vi "Init.vi"(1 "AI Range (V)":cluster{"AImin":dbl, "AImax":dbl}={"AImin"=-10.0, "AImax"=10.0}, 2 "Repetitions":u32, 5 "Pixel Dwell time (s)":dbl format="%#_6p", 7 "Trigger terminal":tag, 9 "AI Channels":tag, 11 "error in":errorcluster, 12 "input terminal configuration":i32(ring)=-1 items=["default"=-1, "RSE"=10083, "NRSE"=10078, "Differential"=10106, "Pseudodifferential"=12529]) -> (4 "AI Task out":refnum<k21>, 15 "error out":errorcluster)   [LabVIEW 2025]
uses:
  <vilib>/DAQmx/create/channels.llb/DAQmx Create Channel (AI-Voltage-Basic).vi
  <vilib>/DAQmx/configure/timing.llb/DAQmx Timing (Sample Clock).vi
  <vilib>/DAQmx/configure/trigger.llb/DAQmx Start Trigger (Digital Edge).vi
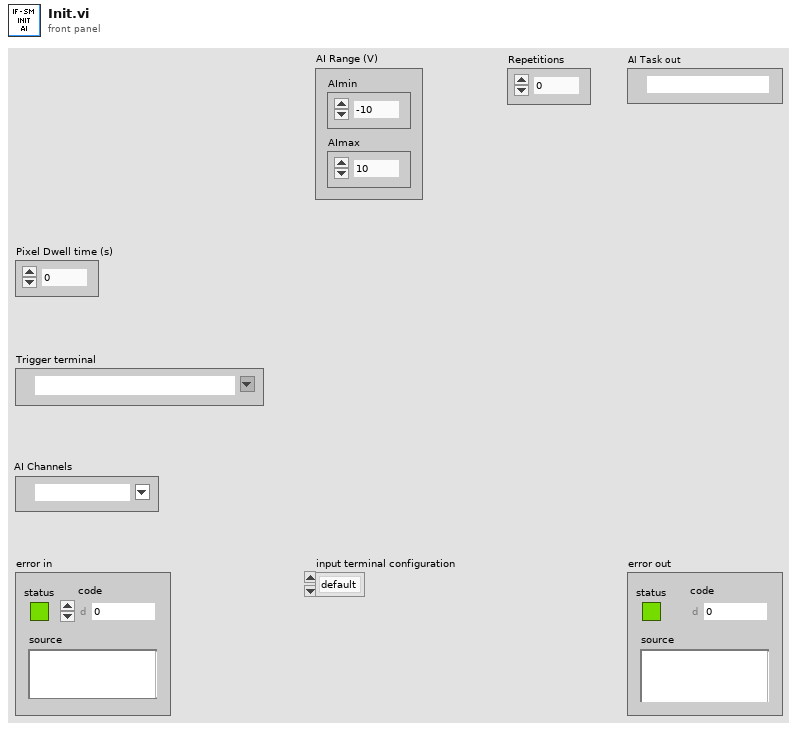
[diagram p1: front panel]
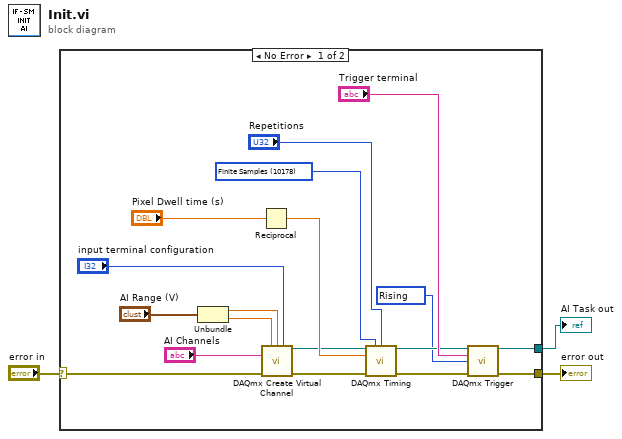
[diagram p0: block diagram]
diagram:
  n1 = case shown="No Error" "error in" {
    selector: "error in" -> [w4 w22]
    tunnel: [w21 w22] -> w3
    tunnel: [w5 _] -> w2
    frame No Error {
      w9 = 10280 items=["Rising"=10280, "Falling"=10171] ("edge")
      w15 = 10178 items=["Finite Samples"=10178, "Continuous Samples"=10123] ("sample mode")
      n2 = Unbundle("AI Range (V)") -> ("AImin"=w7:dbl, "AImax"=w6:dbl)
      n3 = Reciprocal(x="Pixel Dwell time (s)") -> (1/x=w19:dbl)
      n4 = call-poly <vilib>:"DAQmx Create Virtual Channel.vi"("maximum value"=w6, "minimum value"=w7, "input terminal configuration"="input terminal configuration", "physical channels"="AI Channels", "error in"=w4) -> ("task out"=w14:refnum<k21>, "error out"=w13:errorcluster)  [unwired: 9 in]
      n5 = call-poly <vilib>:"DAQmx Timing.vi"("task/channels in"=w14, "sample mode"=w15, "samples per channel"="Repetitions", "rate"=w19, "error in"=w13) -> ("task out"=w11:refnum<k21>, "error out"=w10:errorcluster)  [unwired: 9 in]
      n6 = call-poly <vilib>:"DAQmx Trigger.vi"("task/channels in"=w11, "source"="Trigger terminal", "edge"=w9, "error in"=w10) -> ("task out"=w5:refnum<k21>, "error out"=w21:errorcluster)  [unwired: 10 in]
    }
    frame Error {
    }
  }
  "error out" <- w3
  "AI Task out" <- w2
